vi "Select Plot Group.vi"(8 "error in (no error)":errorcluster, 10 "Plot Group":string, 11 "HistorianCharting in":refnum<class "HistorianCharting.lvclass">) -> (0 "error out":errorcluster, 3 "HistorianCharting out":refnum<class "HistorianCharting.lvclass">)   [LabVIEW 2020, in "VolatusGUIElements.lvlib" / "HistorianCharting.lvclass"]
uses:
  HistorianCharting.lvclass
  HistorianCharting.lvclass/HistorianCharting.ctl
  Volatus/MessageQ/MessageQ.lvclass
  VolatusGUI/Historian Charting Manager/Chart Selection.ctl
  VolatusGUI/Historian Charting Manager/Historian Charting Manager.lvclass
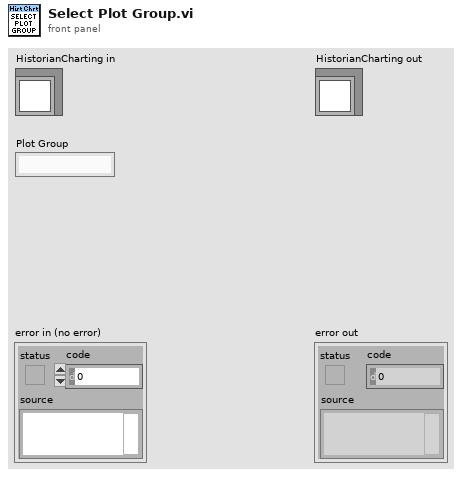
[diagram p1: front panel]
types:
  T1 = typedef "VolatusGUI.lvlib/Historian Charting Manager.lvclass/Chart Selection.ctl" = cluster{"Chart Num":i32, "Plot Group":string}
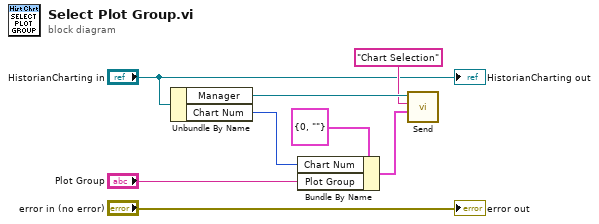
[diagram p0: block diagram]
diagram:
  n1 = Unbundle By Name("HistorianCharting in") -> ("Manager"=w7:refnum<class "MessageQ.lvclass">, "Chart Num"=w4:i32)
  n2 = Bundle By Name(cluster=T1 {"Chart Num"=0, "Plot Group"=""} ("Chart Selection"), "Chart Num"=w4, "Plot Group"="Plot Group") -> (w3:T1)
  n3 = call "Send.vi"("Data"=w3, "ID"="Chart Selection", "MessageQ in"=w7) -> ()  [unwired: 7 in, 2 out]
  "error out" <- "error in (no error)"
  "HistorianCharting out" <- "HistorianCharting in"
